vi "Execute.vi"(8 "error in (no error)":errorcluster, 11 "Simple Actor in":refnum<class "Simple Actor.lvclass">) -> (0 "error out":errorcluster, 3 "Simple Actor out":refnum<class "Simple Actor.lvclass">)   [LabVIEW 2020, in "Simple Actor.lvlib" / "Simple Actor.lvclass"]
uses:
  Simple Actor.lvclass
  Quit Msg/Quit Msg.lvclass
  E:/NI I Program/Actor Intr Demo/Simple Actor/Actor Msg/Actor Msg.lvclass
  Simple Actor.lvclass/Simple Actor.ctl
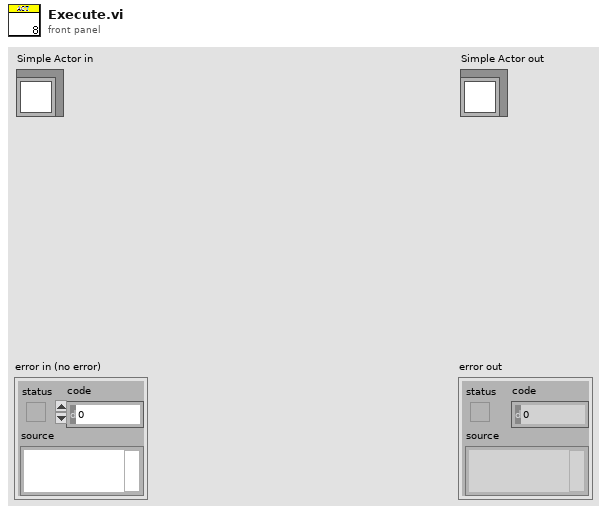
[diagram p1: front panel]
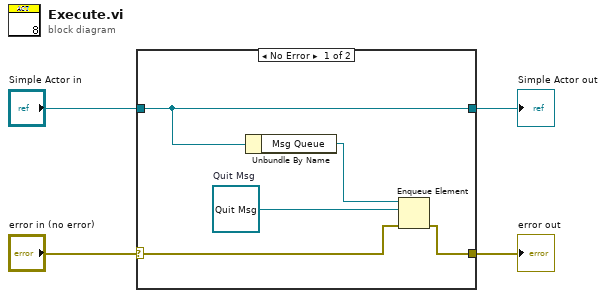
[diagram p0: block diagram]
diagram:
  n1 = case shown="No Error" "error in (no error)" {
    selector: "error in (no error)" -> [w7 w11]
    tunnel: [w6 w11] -> w3
    tunnel: [w8 w10] -> w1
    tunnel: "Simple Actor in" -> [w8 w10]
    frame No Error {
      w5 = refnum<class "Quit Msg.lvclass"> refnum  # Quit Msg
      n2 = Unbundle By Name(w8) -> ("Msg Queue"=w9:refnum<queue>)
      n3 = Enqueue Element(queue=w9, element=w5, error in (no error)=w7) -> (error out=w6:errorcluster)  [unwired: 1 in, 2 out]
    }
    frame Error {
    }
  }
  "error out" <- w3
  "Simple Actor out" <- w1
